vi "get Active VIs.vi"(8 "error in (no error)":errorcluster, 11 "VI Collection in":refnum<class "VI Collection.lvclass">) -> (0 "error out":errorcluster, 2 "Active VI":refnum<vi>[](array[refnum]), 3 "VI Collection out":refnum<class "VI Collection.lvclass">)   [LabVIEW 2014, in "QuickVIew.lvlib" / "VI Collection.lvclass"]
uses:
  VI Collection.lvclass
  VI Collection.lvclass/VI Collection.ctl
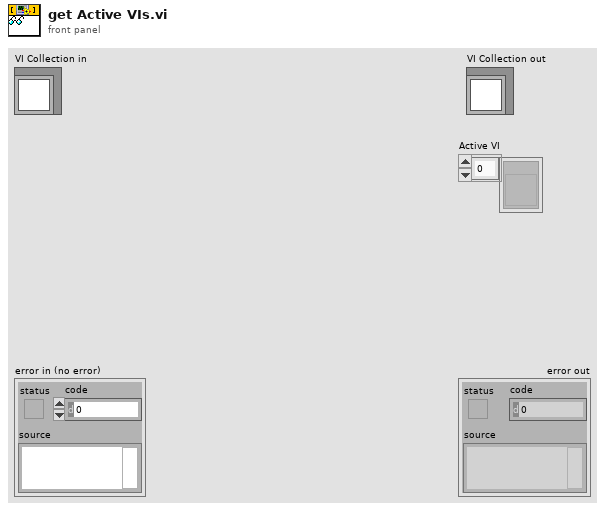
[diagram p1: front panel]
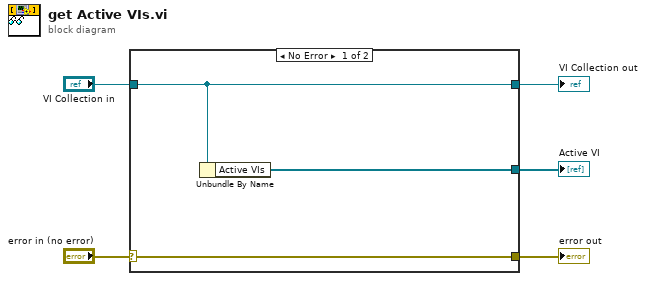
[diagram p0: block diagram]
diagram:
  n1 = case shown="No Error" "error in (no error)" {
    selector: "error in (no error)" -> [w8 w9]
    tunnel: [w8 w9] -> w4
    tunnel: [w6 w10] -> w2
    tunnel: "VI Collection in" -> [w6 w10]
    tunnel: [w7 _] -> w1
    frame No Error {
      n2 = Unbundle By Name(w6) -> ("Active VIs"=w7:refnum<vi>[])
    }
    frame Error {
    }
  }
  "error out" <- w4
  "VI Collection out" <- w2
  "Active VI" <- w1
